vi "Configure Sweep (List).vi"(0 "VISA resource name":refnum<visa-resource-name>, 5 "List Define (0: User Defined)":u16(ring) items=["User Defined", "Preset Default", "Load From Step"], 7 "Frequency Array":dbl[](array[numeric])=[100000.0, 100000.0, 100000.0], 9 "Power Array":dbl[](array[numeric])=[0.0, 0.0, 0.0], 11 "error in (no error)":errorcluster, 12 "Dwell Time Array":dbl[](array[numeric])=[0.002, 0.002, 0.002]) -> (4 "VISA resource name out":refnum<visa-resource-name>, 15 "error out":errorcluster)   [LabVIEW 2018, in "Agilent PSG MXG Series.lvlib"]
doc: "Configrues frequency, amplitude and dwell time for points in the list sweep."
uses:
  Agilent PSG MXG Series.lvlib
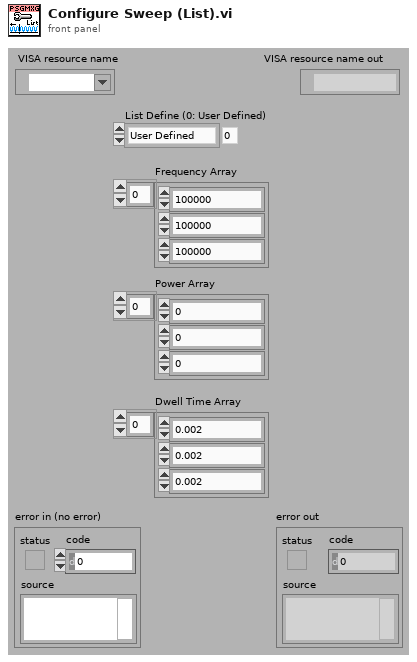
[diagram p1: front panel]
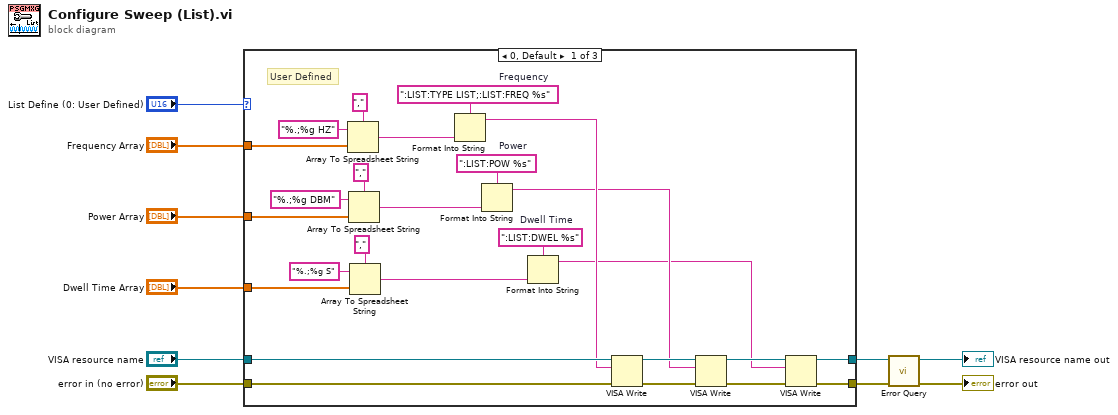
[diagram p0: block diagram]
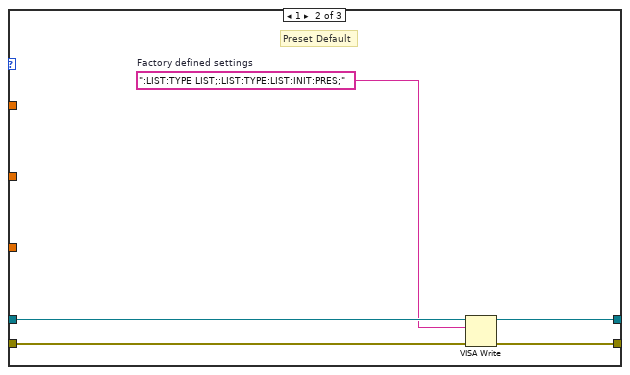
[diagram p2: hidden frame]
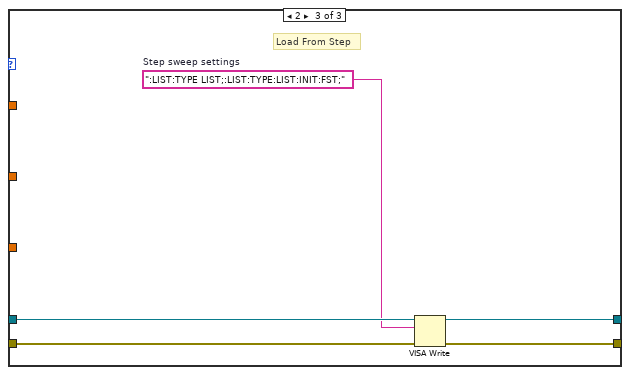
[diagram p3: hidden frame]
diagram:
  n1 = case shown="0, Default" "List Define (0: User Defined)" {
    tunnel: "Frequency Array" -> [w30 _ _]
    tunnel: "Power Array" -> [w28 _ _]
    tunnel: "Dwell Time Array" -> [w27 _ _]
    tunnel: "VISA resource name" -> [w26 w41 w46]
    tunnel: "error in (no error)" -> [w25 w40 w45]
    tunnel: [w15 w39 w43] -> w6
    tunnel: [w14 w38 w42] -> w5
    frame 0, Default {
      w19 = ":LIST:DWEL %s"  # Dwell Time
      w21 = ":LIST:POW %s"  # Power
      w29 = ":LIST:TYPE LIST;:LIST:FREQ %s"  # Frequency
      # "User Defined"
      n2 = Array To Spreadsheet String(delimiter (Tab)=",", array=w30, 3:"%.;%g HZ" ("format string")) -> (spreadsheet string=w13:string)
      n3 = Array To Spreadsheet String(delimiter (Tab)=",", array=w28, 3:"%.;%g DBM" ("format string")) -> (spreadsheet string=w12:string)
      n4 = Array To Spreadsheet String(delimiter (Tab)=",", array=w27, 3:"%.;%g S" ("format string")) -> (spreadsheet string=w11:string)
      n5 = Format Into String(format string=w29, w13) -> (resulting string=w24:string)  [unwired: 2 in, 1 out]
      n6 = Format Into String(format string=w21, w12) -> (resulting string=w20:string)  [unwired: 2 in, 1 out]
      n7 = Format Into String(format string=w19, w11) -> (resulting string=w16:string)  [unwired: 2 in, 1 out]
      n8 = VISA Write(VISA resource name=w26, write buffer=w24, error in (no error)=w25) -> (VISA resource name out=w23:refnum<visa-resource-name>, error out=w22:errorcluster)  [unwired: 1 out]
      n9 = VISA Write(VISA resource name=w23, write buffer=w20, error in (no error)=w22) -> (VISA resource name out=w18:refnum<visa-resource-name>, error out=w17:errorcluster)  [unwired: 1 out]
      n10 = VISA Write(VISA resource name=w18, write buffer=w16, error in (no error)=w17) -> (VISA resource name out=w15:refnum<visa-resource-name>, error out=w14:errorcluster)  [unwired: 1 out]
    }
    frame 1 {
      w37 = ":LIST:TYPE LIST;:LIST:TYPE:LIST:INIT:PRES;"  # Factory defined settings
      # "Preset Default"
      n11 = VISA Write(VISA resource name=w41, write buffer=w37, error in (no error)=w40) -> (VISA resource name out=w39:refnum<visa-resource-name>, error out=w38:errorcluster)  [unwired: 1 out]
    }
    frame 2 {
      w44 = ":LIST:TYPE LIST;:LIST:TYPE:LIST:INIT:FST;"  # Step sweep settings
      # "Load From Step"
      n12 = VISA Write(VISA resource name=w46, write buffer=w44, error in (no error)=w45) -> (VISA resource name out=w43:refnum<visa-resource-name>, error out=w42:errorcluster)  [unwired: 1 out]
    }
  }
  n13 = call "Error Query.vi"("error in (no error)"=w5, "VISA resource name"=w6) -> ("error out"=→"error out":errorcluster, "VISA resource name out"=→"VISA resource name out":refnum<visa-resource-name>)  [unwired: 8 out]
